vi "TestPublishRate.vi"(8 "error in (no error)":errorcluster, 11 "TestPublishRate In":refnum<class "TestPublishRate.lvclass">) -> (0 "error out":errorcluster, 3 "TestPublishRate Out":refnum<class "TestPublishRate.lvclass">)   [LabVIEW 2017, in "TestPublishRate.lvclass"]
uses:
  TestPublishRate.lvclass
  Source/Framework/IViewModel/IViewModel/IViewModel.lvclass
  C:/Git/mva-framework/Source/Framework/IObserver/IObserver/IObserver.lvclass
  C:/Git/mva-framework/Source/Framework/IViewManager/IViewManager/IViewManager.lvclass
  C:/Program Files (x86)/National Instruments/LabVIEW 2017/vi.lib/ActorFramework/Actor/Actor.lvclass
  Source/Framework/IViewable/IViewable/IViewable.lvclass
  Doubles/TestModelFastPublish/TestModelFastPublish.lvclass
  C:/Git/mva-framework/Source/Framework/IModel/IModel/IModel.lvclass
  Source/Framework/Mediator/Mediator/Mediator.lvclass
  C:/Git/mva-framework/Source/Framework/IMediator/IMediator/IMediator.lvclass
  Source/Framework/IObserver/IObserver/IObserver.lvclass/IObserver.ctl
  Source/Framework/IMediator/IMediator/IMediator.lvclass/IMediator.ctl
  Source/Framework/IViewManager/IViewManager Messages/Launch Nested Views Msg/Launch Nested Views Msg.lvclass/Launch Nested Views Msg.ctl
  Source/Framework/IViewModel/IViewModel/IViewModel.lvclass/IViewModel.ctl
  Source/Framework/IViewManager/IViewManager/IViewManager.lvclass/IViewManager.ctl
  Source/Framework/SubscriptionPolicy/ValueChangeSubscription/ValueChangeSubscription.lvclass/ValueChangeSubscription.ctl
  Source/Framework/IMediator/SubscriptionRequest/SubscriptionRequest.lvclass/SubscriptionRequest.ctl
  Source/Framework/IObserver/IObserver Messages/Subscribe Msg/Subscribe Msg.lvclass/Subscribe Msg.ctl
  <vilib>/ActorFramework/Message Enqueuer/Message Enqueuer.lvclass/Message Enqueuer.ctl
  gpm_packages/@cs/transport/Source/Concrete/QueueTransport/QueueTransport.lvclass/QueueTransport.ctl
  <vilib>/ActorFramework/Stop Msg/Stop Msg.lvclass/Stop Msg.ctl
  <vilib>/Analysis/baseanly.llb/Mean (DBL).vi
  36929478-dcdb-4b78-a758-5699a0901173.vi
  <vilib>/ActorFramework/Message Enqueuer/Enqueue.vi
  <vilib>/ActorFramework/Message Enqueuer/Enqueue Critical.vi
  Source/Framework/IObserver/IObserver/Configure Observer Logging.vi
  Source/Framework/IViewModel/IViewModel/Write Startup Model-View Configuration.vi
  Source/Framework/IMediator/IMediator/Configure Mediator.vi
  Source/Framework/IViewManager/IViewManager Messages/Launch Nested Views Msg/Pack Launch Nested Views Msg.vi
  Source/Framework/IViewManager/IViewManager/Write Startup Launch Nested Views Msg.vi
  gpm_packages/@cs/transport/Source/Concrete/QueueTransport/QueueTransport.lvclass
  C:/Git/mva-framework/gpm_packages/@cs/transport/Source/ITransport/ITransport.lvclass
  Source/Framework/SubscriptionPolicy/ValueChangeSubscription/ValueChangeSubscription.lvclass
  C:/Git/mva-framework/Source/Framework/IMediator/ISubscriptionPolicy/ISubscriptionPolicy.lvclass
  Source/Framework/IObserver/IObserver Messages/Subscribe Msg/Subscribe Msg.lvclass
  C:/Program Files (x86)/National Instruments/LabVIEW 2017/vi.lib/ActorFramework/Message/Message.lvclass
  <vilib>/ActorFramework/Stop Msg/Stop Msg.lvclass
  <vilib>/ActorFramework/Message Priority Queue/Priority Enqueue.vi
  <vilib>/Utility/error.llb/Error Cluster From Error Code.vi
  Source/Framework/IViewManager/IViewManager Messages/Launch Nested Views Msg/Launch Nested Views Msg.lvclass
  Source/Framework/IViewable/IApplicationStyle/IApplicationStyle.lvclass
  gpm_packages/@cs/event-logger/Source/Composed Log/LoggerReference/LoggerReference.lvclass
  gpm_packages/@cs/event-logger/Source/Text File Sink/Text File Sink.lvclass
  Source/Framework/IMediator/IMediatorBusMonitor/IMediatorBusMonitor.lvclass
  Source/Framework/IMediator/SubscriptionRequest/SubscriptionRequest.lvclass
  <vilib>/ActorFramework/Actor/Actor.lvclass
  Source/Framework/IMediator/ISubscriptionPolicy/ISubscriptionPolicy.lvclass
  <vilib>/Analysis/NI_AALBase.lvlib
panel:
  out "Avg Transit Time":dbl format="%#_3p"
  out "Iteration":i32
  out "Transmission Times":dbl[](graph)
  out "Actual Publish Period":dbl[](graph)
  # "0.5 sec final sample time typical"
  # "100us or less"
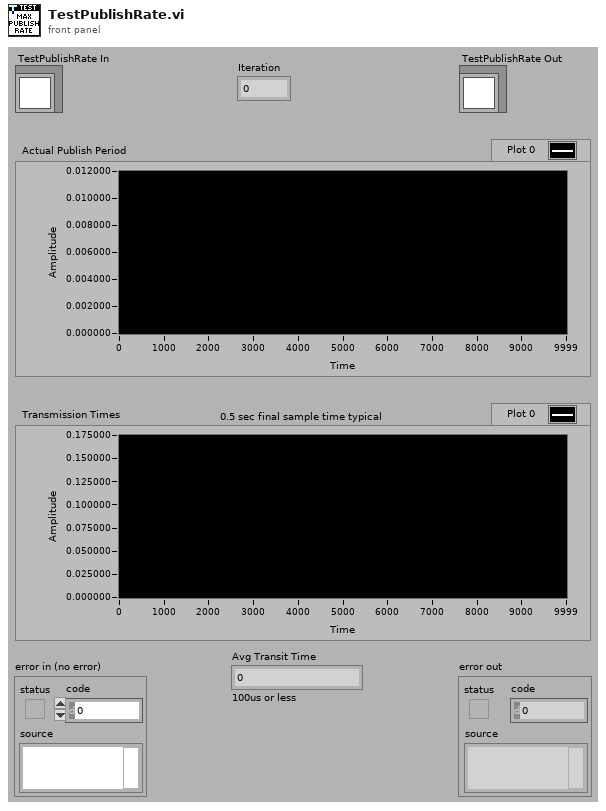
[diagram p1: front panel]
types:
  T1 = typedef "IMediator.lvlib/ISubscriptionPolicy.lvclass/ISubscriptionPolicy Reference.ctl" = refnum<data-value>
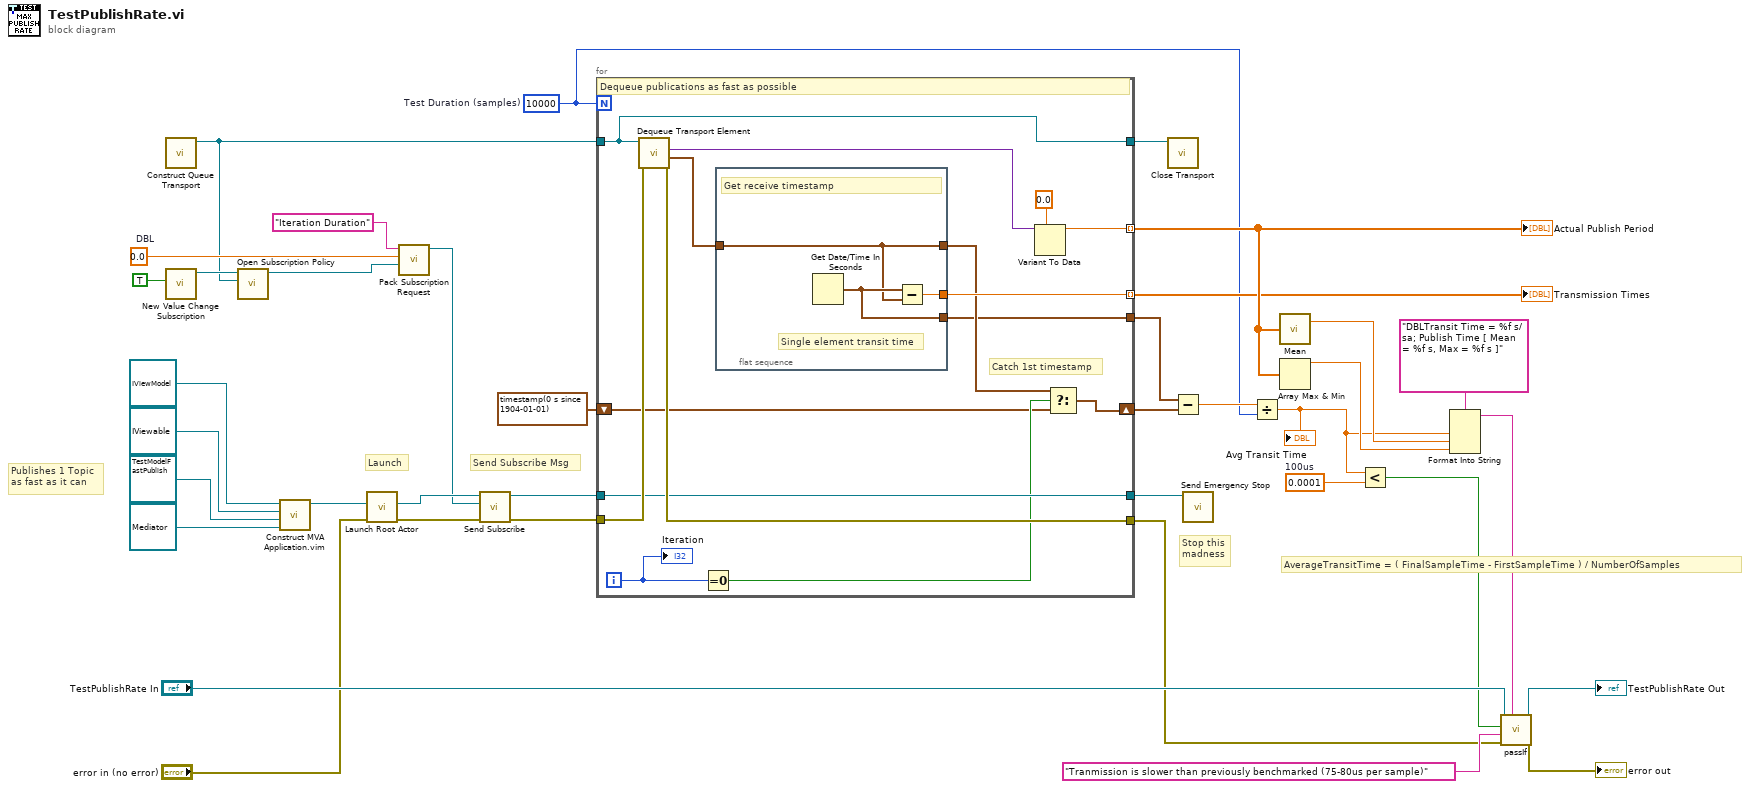
[diagram p0: block diagram]
diagram:
  w8 = 0.0001  # 100us
  w4 = 10000  # Test Duration (samples)
  w22 = 0.0  # DBL
  # "Publishes 1 Topic\nas fast as it can"
  # "AverageTransitTime = ( FinalSampleTime - FirstSampleTime ) / NumberOfSamples"
  # "Stop this\nmadness"
  # "Send Subscribe Msg"
  # "Launch"
  n1 = call "Construct Queue Transport.vi"() -> ("QueueTransport"=w3:refnum<class "QueueTransport.lvclass">)  [unwired: 10 in, 1 out]
  n2 = call "New Value Change Subscription.vi"("Ignore Past Updates? (F)"=TRUE) -> ("ValueChangeSubscription Out"=w29:refnum<class "ValueChangeSubscription.lvclass">)  [unwired: 10 in]
  n3 = call "Open Subscription Policy.vi"("Transport"=w3, "SubscriptionPolicy"=w29) -> ("Subscription Policy"=w1:T1)  [unwired: 8 in, 1 out]
  n4 = call "Construct MVA Application.vim"("Mediator Type"=refnum<class "Mediator.lvclass"> refnum ("Mediator"), "Model Type"=refnum<class "TestModelFastPublish.lvclass"> refnum ("Model"), "Startup View Configuration"=refnum<class "IViewable.lvclass"> refnum, "IViewModel In"=refnum<class "IViewModel.lvclass"> refnum) -> ("IViewModel Out"=w31:refnum<class "IViewModel.lvclass">)  [unwired: 7 in]
  n5 = call <vilib>:"Launch Root Actor.vi"("error in (no error)"="error in (no error)", "Actor"=w31) -> ("error out"=w25:errorcluster, "Actor's Enqueuer"=w30:refnum<class "Message Enqueuer.lvclass">)  [unwired: 8 in]
  n6 = call "Pack Subscription Request.vi"("Subscription Policy"=w1, "Type"=w22, "Datum Name"="Iteration Duration" ("Topic Name")) -> ("SubscriptionRequest"=w27:refnum<class "SubscriptionRequest.lvclass">)  [unwired: 8 in]
  n7 = call "Send Subscribe.vi"("error in (no error)"=w25, "SubscriptionRequest"=w27, "Message Enqueuer"=w30) -> ("error out"=w24:errorcluster, "Message Enqueuer out"=w26:refnum<class "Message Enqueuer.lvclass">)  [unwired: 7 in]
  n8 = for {
    N: w4 -> [_]
    tunnel: w26 -> [w49]
    tunnel: w24 -> [w53]
    tunnel: w3 -> [w39]
    tunnel: [w51] -> w18 mode=indexing
    tunnel: [w50] -> w15 mode=indexing
    tunnel: [w52] -> w5
    tunnel: [w49] -> w17
    tunnel: [w39] -> w16
    shift-right: [w48] -> w12
    shift-left: timestamp(0 s since 1904-01-01) ("Publication Time") -> [w44]
    tunnel: [w43] -> w13
    i -> [w46]
    # "Catch 1st timestamp"
    # "Dequeue publications as fast as possible"
    n9 = call "Dequeue Transport Element.vi"("error in (no error)"=w53, "QueueTransport"=w39) -> ("error out"=w52:errorcluster, "Publication Time"=w41:timestamp, "Data"=w40:variant)  [unwired: 6 in, 1 out]
    n10 = Equal To 0?(x=w46) -> (x = 0?=w45:bool)
    n11 = flat-sequence {
      tunnel: [w56] -> w50
      tunnel: [w54] -> w47
      tunnel: [w55] -> w43
      tunnel: w41 -> [w54]
      frame #0 {
        # "Single element transit time"
        # "Get receive timestamp"
        n12 = Get Date/Time In Seconds() -> (seconds since 1Jan1904=w55:timestamp)
        n13 = Subtract(x=w55, y=w54) -> (x-y=w56:dbl)
      }
    }
    n14 = Variant To Data(type=0.0, Variant=w40) -> (data=w51:dbl)  [unwired: 1 in, 1 out]
    n15 = Select(t=w47, s=w45, f=w44) -> (s? t:f=w48:timestamp)
    "Iteration" <- w46
  }
  "Actual Publish Period" <- w18
  "Transmission Times" <- w15
  n16 = call-dynamic "Close Transport.vi"("QueueTransport"=w16) -> ()  [unwired: 10 in, 1 out]
  n17 = Subtract(x=w13, y=w12) -> (x-y=w11:dbl)
  n18 = call <vilib>:"Send Emergency Stop.vi"("Message Enqueuer"=w17) -> ()  [unwired: 10 in, 1 out]
  n19 = Divide(x=w11, y=w4) -> (x/y=w9:dbl)
  "Avg Transit Time" <- w9
  n20 = call-poly <vilib>:"Mean.vi"("X"=w18) -> ("mean"=w20:dbl)  [unwired: 1 out]
  n21 = Array Max & Min(array=w18) -> (max value=w19:dbl)  [unwired: 3 out]
  n22 = Less?(x=w9, y=w8) -> (x < y?=w7:bool)
  n23 = Format Into String(format string="DBLTransit Time = %f s/sa; Publish Time [ Mean = %f s, Max = %f s ]", w9, w20, w19) -> (resulting string=w10:string)  [unwired: 2 in, 1 out]
  n24 = call-dynamic "passIf.vi"("custom report message (\"\")"=w10, "error in (no error)"=w5, "message (\"\")"="Tranmission is slower than previously benchmarked (75-80us per sample)" ("message (\"\")"), "pass"=w7, "TestCase in"="TestPublishRate In") -> ("error out"=→"error out":errorcluster, "TestCase out"=→"TestPublishRate Out":refnum<class "TestPublishRate.lvclass">)  [unwired: 5 in]
